vi "save.vi"(8 "Error In":errorcluster, 10 "fileName":string, 11 "QPixmap In":refnum<class "QPixmap.lvclass">) -> (0 "Error Out":errorcluster, 2 "Value":bool, 3 "QPixmap Out":refnum<class "QPixmap.lvclass">)   [LabVIEW 2014, in "QPixmap.lvclass"]
doc: "LabVIEW-specific documentation is not yet available. See <b>https://doc.qt.io/qt-5/qpixmap.html#save</b>"
uses:
  QPixmap.lvclass
  LQ Core/LQSerialData/LQSerialData.lvclass/LQSerialData.ctl
  LQ Core/LQ Core.lvlib
  LQ Core/LQSerialData/LQSerialData.lvclass
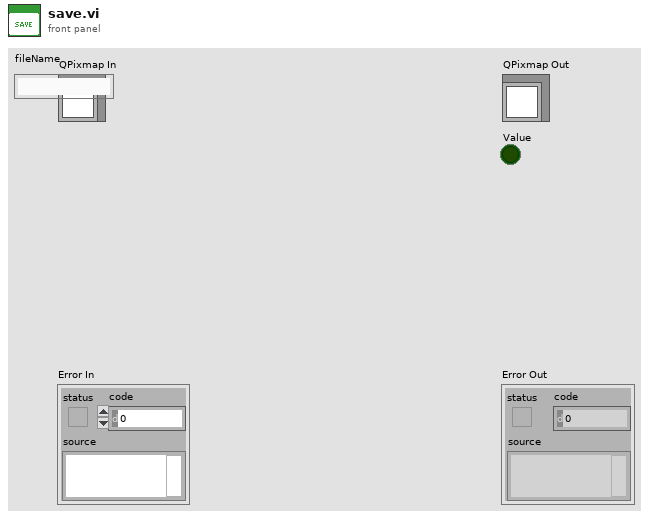
[diagram p1: front panel]
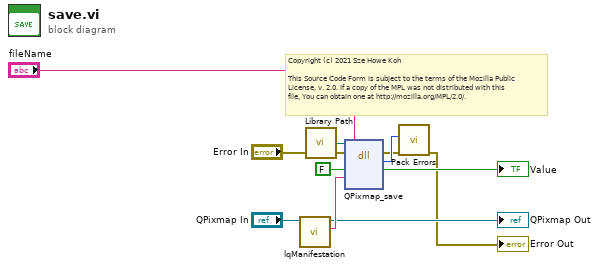
[diagram p0: block diagram]
diagram:
  # "Copyright (c) 2021 Sze Howe Koh\n\nThis Source Code Form is subject to the terms of the Mozilla Public\nLicense, v. 2.0. If a copy of the MPL was not distributed with this\nfile, You can obtain one at http://mozilla.org/MPL/2.0/."
  n1 = call "lqManifestation.vi"("LQSerialData in"="QPixmap In") -> ("Manifestation"=w8:string, "LQSerialData out"=→"QPixmap Out":refnum<class "QPixmap.lvclass">)  [unwired: 9 in]
  n2 = call "Library Path.vi"() -> ("Library Path"=w5:path)
  n3 = dll-call lib="?" fn="QPixmap_save"(path in=w5, error in="Error In", "_retVal"=FALSE, "_instance"=w8, "fileName"="fileName") -> (error out=w3:errorcluster, w4:i32, "_retVal"=→"Value":bool)  [unwired: 3 in, 1 out]
  n4 = call "Pack Errors.vi"("Error In"=w3, "Error Code"=w4) -> ("Error Out"=→"Error Out":errorcluster)  [unwired: 9 in]
